vi "MIMIC Commands Rev 5.vi"(6 "MIMIC HOST COMMAND":T2(ring)=enum."Read Serial Number", 8 "Input String Data Array":string[](array[string])=["1"], 9 "HWHSflag":bool, 10 "wait (ms)":u32=500, 11 "VISA resource name":refnum<visa-resource-name>="COM5") -> (0 "error out":errorcluster={"status"=FALSE, "code"=1073676294, "source"="VISA Read in MIMIC RecvCommand.vi->MIMIC Commands Rev 2.vi"}, 1 "Receive_buffer":u8[](array[numeric]) format="%x", 2 "Receive_Unpacked_Data":T1)   [LabVIEW 2014]
panel:
  out "GUID":string
  out "Array":u8[](array[numeric])
  out "TimeToDecode":u16
  out "VISA resource name OUT":refnum<visa-resource-name>="COM5"
  out "hex integer string":string[](array[string])=["4", "D0", "0", "0", "FF", "2C"]
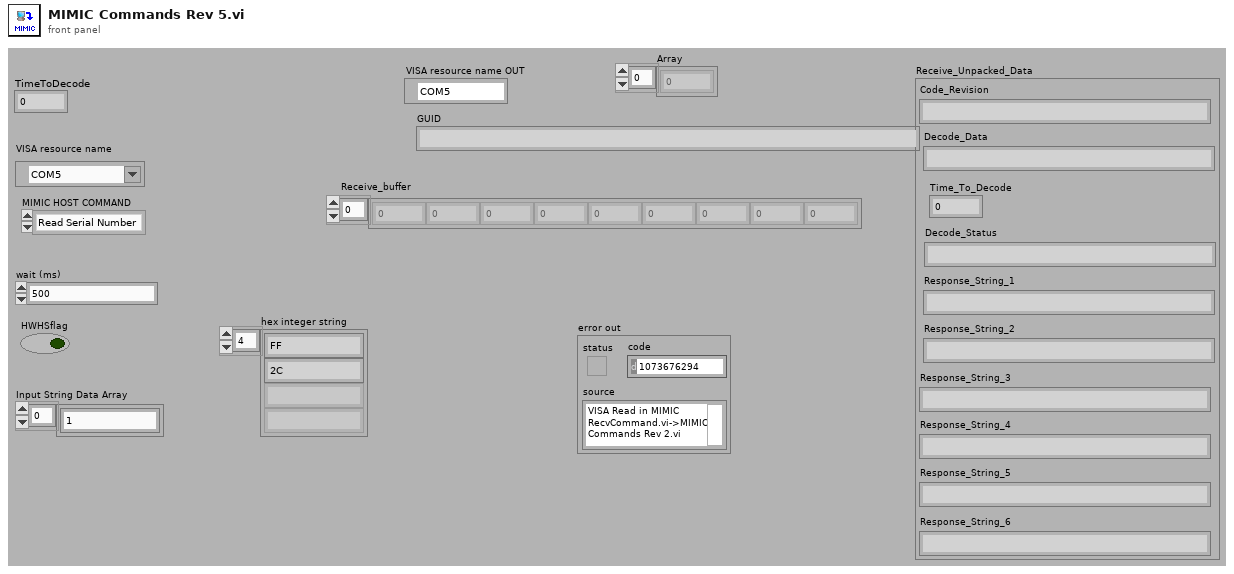
[diagram p1: front panel]
types:
  T1 = cluster{"Code_Revision":string, "Decode_Data":string, "Decode_Status":string, "Response_String_1":string, "Response_String_2":string, "Response_String_3":string, "Response_String_4":string, "Response_String_5":string, "Response_String_6":string, "Time_To_Decode":u16}
  T2 = enum16{"Enter FAT", "Beeper Control", "LED Off", "LED On", "Image Mode", "Start Session", "Stop Session", "Change Buadrate", "Auto Exposure", "Set Manual Exposure", "Read BT Address", "Store BT Address", "Pairing Command", "Query Paired Address", "Pairing Status", "Un-Pairing", "Set Illumination", "Trigger", "Set Defaults", "Imager Time To Decode Test", "Battery Off", "Battery Charge Control", "Read Battery Voltage", "Read Battery Temperature", "Software Version", "StoreFeatureSet", "ReadFeatureSet", "Store Model Number", "Read Model Number", "Store Manufacturing Date", "Read Manufacturing Date", "Store Service Date", "Read Service Date", "Store Serial Number", "Read Serial Number", "Exit FAT", "Read GUID", "Cable Auto ID", "Store RSM 627", "Read RSM 627", "Hall Effect switch", "Store GUID ", "Param Send"}
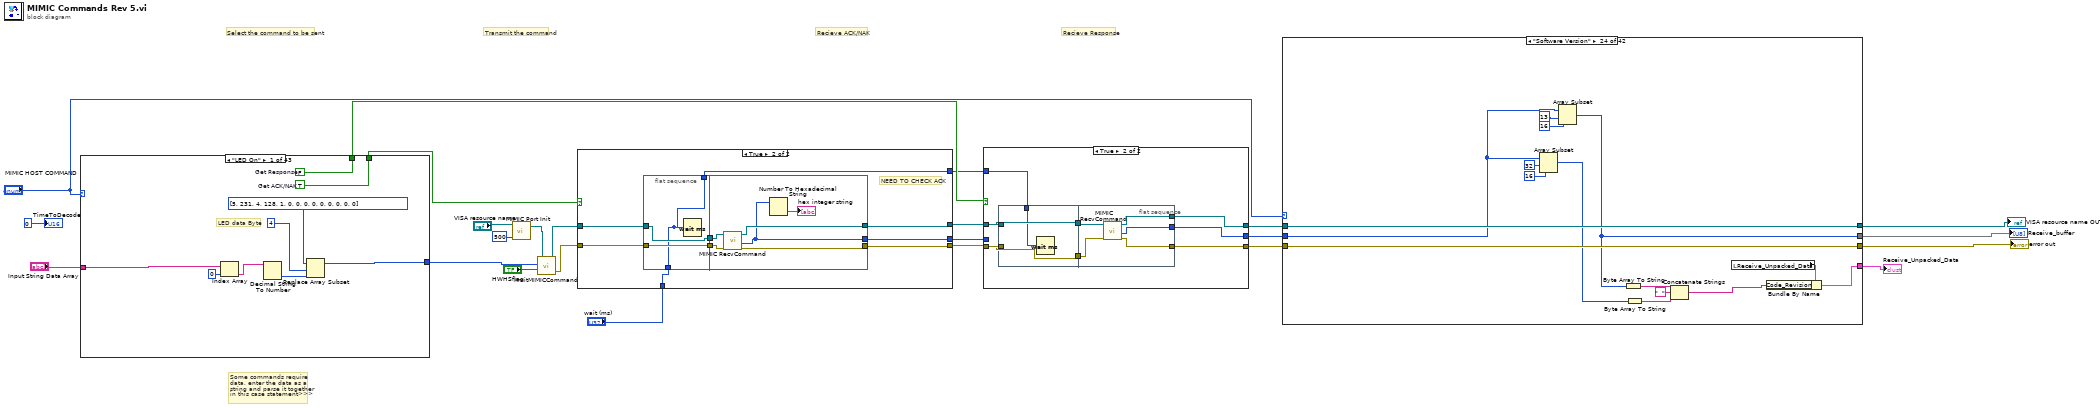
[diagram p0: block diagram]
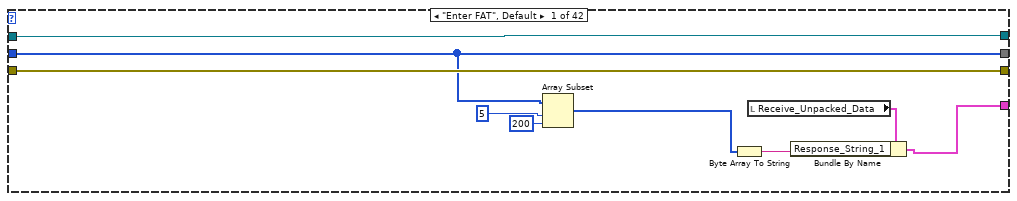
[diagram p2: hidden frame]
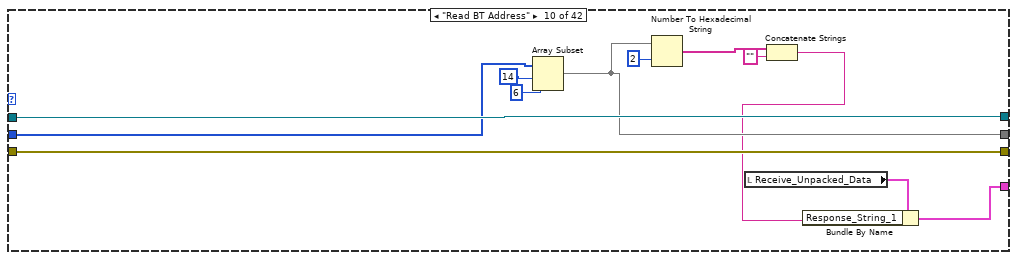
[diagram p11: hidden frame]
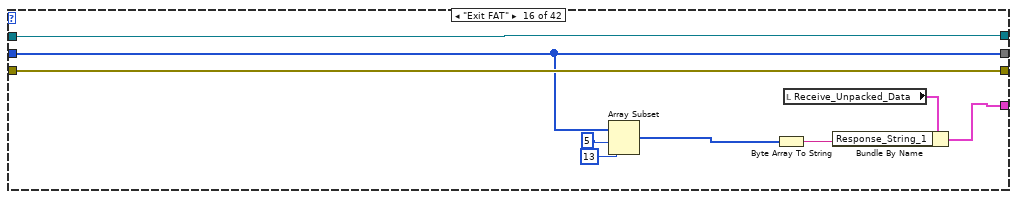
[diagram p17: hidden frame]
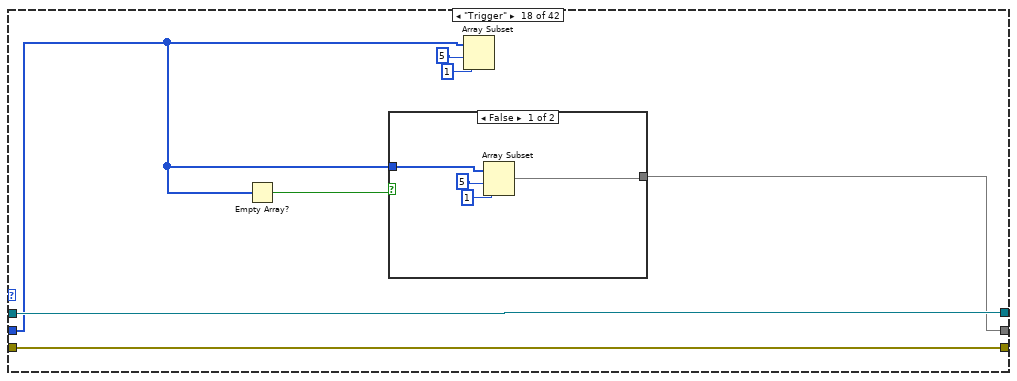
[diagram p19: hidden frame]
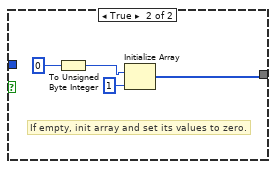
[diagram p20: hidden frame]
diagram:
  # "Transmit the command"
  # "Recieve Response"
  # "Recieve ACK/NAK"
  # "Select the command to be sent"
  # "Some commands require\ndata, enter the data as a\nstring and parse it together\nin this case statement>>>"
  n1 = case shown="\"LED On\"" "MIMIC HOST COMMAND" {
    tunnel: "Input String Data Array" -> [w33 w34 _ w45 _ _ _ w63 w79 w89 w104 w117 _ _ _ _ _ w141 _ _ _ w161 _ _ _ w178 _ w188 _ _ _ w214 _ w226 _ _ _ _ _ _ _ _ _]
    tunnel: [w27 w38 u8[] [5, 161, 4, 128, 16, 0, 0, 0, 0, 0, 0, 0, 0, 0] w46 u8[] [4, 228, 4, 0, 0, 0, 0, 0, 0, 0, 0, 0, 0, 0] u8[] [4, 228, 4, 0, 0, 0, 0, 0, 0, 0, 0, 0, 0, 0] u8[] [7, 215, 4, 0, 4, 11, 0, 255, 15, 0, 0, 0, 0, 0] w64 w73 w87 w102 w116 u8[] [16, 161, 4, 128, 16, 0, 0, 0, 0, 0, 0, 0, 0, 0] u8[] [5, 161, 4, 128, 16, 0, 0, 0, 0, 0, 0, 0, 0, 0] u8[] [4, 200, 4, 128, 0, 0, 0, 0, 0, 0, 0, 0, 0, 0] u8[] [5, 161, 4, 128, 25, 0, 0, 0, 0, 0, 0, 0, 0, 0] u8[] [7, 161, 4, 128, 66, 2, 29, 0, 0, 0, 0, 0, 0, 0] w140 u8[] [6, 161, 4, 128, 45, 2, 0, 0, 0, 0, 0, 0, 0, 0] u8[] [7, 161, 4, 128, 48, 19, 136, 0, 0, 0, 0, 0, 0, 0] u8[] [5, 161, 4, 128, 60, 0, 0, 0, 0, 0, 0, 0, 0, 0] w160 u8[] [7, 161, 4, 128, 66, 117, 48, 0, 0, 0, 0, 0, 0, 0] u8[] [7, 161, 4, 128, 66, 117, 49, 0, 0, 0, 0, 0, 0, 0] u8[] [7, 161, 4, 128, 66, 78, 41, 0, 0, 0, 0, 0, 0, 0] w180 u8[] [7, 161, 4, 128, 66, 2, 194, 0, 0, 0, 0, 0, 0, 0] w193 u8[] [7, 161, 4, 128, 66, 2, 21, 0, 0, 0, 0, 0, 0, 0] w207 u8[] [7, 161, 4, 128, 66, 2, 23, 0, 0, 0, 0, 0, 0, 0] w219 u8[] [7, 161, 4, 128, 66, 2, 24, 0, 0, 0, 0, 0, 0, 0] w231 u8[] [7, 161, 4, 128, 66, 2, 22, 0, 0, 0, 0, 0, 0, 0] u8[] [5, 161, 4, 128, 54, 254, 160, 0, 0, 0, 0, 0, 0, 0] u8[] [5, 161, 4, 128, 84, 0, 0, 0, 0, 0, 0, 0, 0, 0] u8[] [5, 161, 4, 128, 47] w246 u8[] [5, 161, 4, 128, 110] u8[] [10, 161, 4, 128, 69, 2, 115, 66, 7, 2] u8[] [6, 161, 4, 128, 45, 1, 0, 0, 0, 0, 0, 0, 0, 0] u8[] [7, 161, 4, 128, 66, 2, 115]] -> w19
    tunnel: [w26 w36 w43 w47 w55 w58 w60 w65 w80 w90 w105 w123 w126 w128 w131 w135 w139 w143 w150 w154 w157 w158 w169 w172 w174 w183 w186 w192 w197 w206 w211 w218 w222 w229 w234 w238 w242 w243 w251 w253 w256 w259 w263] -> w21
    tunnel: [w25 w37 w42 w48 w56 w59 w61 w66 w81 w91 w106 w124 w127 w129 w132 w134 w138 w142 w151 w153 w156 w159 w168 w171 w173 w182 w185 w191 w198 w205 w210 w217 w223 w230 w235 w237 w241 w244 w252 w254 w257 w260 w262] -> w23
    frame "LED On" {
      w26 = FALSE  # Get Response
      w25 = TRUE  # Get ACK/NAK
      # "LED data Byte"
      n2 = Index Array(array=w33, index=0) -> (element=w32:string)
      n3 = Decimal String To Number(string=w32) -> (number=w31:i32)  [unwired: 2 in, 1 out]
      n4 = Replace Array Subset(array=u8[] [5, 231, 4, 128, 1, 0, 0, 0, 0, 0, 0, 0, 0, 0], new element=w31, index=4) -> (w27:u8[])
    }
    frame "Beeper Control" {
      w36 = FALSE  # Get Response
      w37 = FALSE  # Get ACK/NAK
      # "Beeper data Byte"
      n5 = Decimal String To Number(string=w34, offset=0) -> (number=w41:i32[])  [unwired: 1 in, 1 out]
      n6 = Replace Array Subset(array=u8[] [5, 230, 4, 128, 0, 0, 0, 0, 0, 0, 0, 0, 0, 0], new element=w41, index=4) -> (w38:u8[])
    }
    frame "Enter FAT" {
      w43 = TRUE  # Get Response
      w42 = TRUE  # Get ACK/NAK
      # "Enter FAT command:\n0x05:0xA1:0x40:0x80:0x10"
    }
    frame "Image Mode" {
      w47 = FALSE  # Get Response
      w48 = TRUE  # Get ACK/NAK
      # "Image Mode Byte:\n00: Decode\n01: SnapShot\n02: Video\n03: Last Decode\n04: las No Decode"
      n7 = Index Array(array=w45, index=0) -> (element=w53:string)
      n8 = Decimal String To Number(string=w53) -> (number=w52:i32)  [unwired: 2 in, 1 out]
      n9 = Replace Array Subset(array=u8[] [5, 247, 4, 128, 0, 0, 0, 0, 0, 0, 0, 0, 0, 0], new element=w52, index=4) -> (w46:u8[])
    }
    frame "Start Session" {
      w55 = FALSE  # Get Response
      w56 = TRUE  # Get ACK/NAK
      # "Start Session"
    }
    frame "Stop Session" {
      w58 = FALSE  # Get Response
      w59 = TRUE  # Get ACK/NAK
      # "Start Session"
    }
    frame "Change Buadrate" {
      w60 = FALSE  # Get Response
      w61 = FALSE  # Get ACK/NAK
      # "Enter FAT command:\n06: 9600\n08: 38400\n0A: 57600\n0B:115200\n0C:230400"
    }
    frame "Auto Exposure" {
      w65 = FALSE  # Get Response
      w66 = TRUE  # Get ACK/NAK
      # "Auto Exposure:\n00:Disabled\n01: Enabled"
      n10 = Index Array(array=w63, index=0) -> (element=w71:string)
      n11 = Decimal String To Number(string=w71) -> (number=w70:i32)  [unwired: 2 in, 1 out]
      n12 = Replace Array Subset(array=u8[] [8, 198, 4, 0, 255, 240, 41, 0, 0, 0, 0, 0, 0, 0], new element=w70, index=7) -> (w64:u8[])
    }
    frame "Set Manual Exposure" {
      w80 = FALSE  # Get Response
      w81 = TRUE  # Get ACK/NAK
      # "Image Mode Byte:\n00: Decode\n01: SnapShot\n02: Video\n03: Last Decode\n04: las No Decode"
      n13 = Index Array(array=w79, index=0) -> (element=w85:string)
      n14 = Decimal String To Number(string=w85, default (0L)=u16 0 ("default (0 I32)")) -> (number=w78:u16)  [unwired: 1 in, 1 out]
      n15 = Split Number(x=w78) -> (hi(x)=w76:u8, lo(x)=w75:u8)
      n16 = Replace Array Subset(array=u8[] [10, 198, 4, 0, 255, 244, 241, 55, 0, 0, 0, 0, 0, 0], new element=w76, index=8) -> (w72:u8[])
      n17 = Replace Array Subset(array=w72, new element=w75, index=9) -> (w73:u8[])
    }
    frame "Store BT Address" {
      w90 = FALSE  # Get Response
      w91 = TRUE  # Get ACK/NAK
      # "Store BT command:\n0x16, 0xA1, 0x04, 0x80, 0x45, 0x02, 0x1D, 0x41, 0x07, 0x42, 0x00, 0x06, 0x00, 0x00, \n\t\t\t\t\t\t\t\t\t\t0x00, 0x00, 0x00, 0x00, 0x00, 0x00,0x00, 0x00, 0xFF, 0xFF};"
      n18 = for {
        N: 6 -> [_]
        tunnel: w89 -> [w100]
        tunnel: [w95] -> w87
        i -> [w97]
        n19 = Index Array(array=w100, index=w97) -> (element=w94:string)
        n20 = Add(x=14 ("index"), y=w97) -> (x+y=w98:i32)
        n21 = Hexadecimal String To Number(string=w94, offset=0) -> (number=w92:u32)  [unwired: 1 in, 1 out]
        n22 = local read "Array"() -> (w96:u8[])
        n23 = Replace Array Subset(array=w96, new element=w92, index=w98) -> (w95:u8[])
        n24 = local write "Array"(w95) -> ()
      }
      "Array" <- u8[] [22, 161, 4, 128, 69, 2, 29, 65, 7, 66, 0, 6, 0, 0, 0, 0, 0, 0, 0, 0, 255, 255, 255, 0, 0, 0]
    }
    frame "Param Send" {
      w105 = FALSE  # Get Response
      w106 = TRUE  # Get ACK/NAK
      # "Store BT command:\n0x16, 0xA1, 0x04, 0x80, 0x45, 0x02, 0x1D, 0x41, 0x07, 0x42, 0x00, 0x06, 0x00, 0x00, \n\t\t\t\t\t\t\t\t\t\t0x00, 0x00, 0x00, 0x00, 0x00, 0x00,0x00, 0x00, 0xFF, 0xFF};"
      n25 = for {
        N: 6 -> [_]
        tunnel: w104 -> [w115]
        tunnel: [w110] -> w102
        i -> [w112]
        n26 = Index Array(array=w115, index=w112) -> (element=w109:string)
        n27 = Add(x=14 ("index"), y=w112) -> (x+y=w113:i32)
        n28 = Hexadecimal String To Number(string=w109, offset=0) -> (number=w107:u32)  [unwired: 1 in, 1 out]
        n29 = local read "Array"() -> (w111:u8[])
        n30 = Replace Array Subset(array=w111, new element=w107, index=w113) -> (w110:u8[])
        n31 = local write "Array"(w110) -> ()
      }
      n32 = local write "Array"(u8[] [22, 161, 4, 128, 69, 2, 29, 65, 7, 66, 0, 6, 0, 0, 0, 0, 0, 0, 0, 0, 255, 255, 255, 0, 0, 0]) -> ()
    }
    frame "Pairing Command" {
      w123 = TRUE  # Get Response
      w124 = FALSE  # Get ACK/NAK
      # "Pairing  command:\n10 9E 04 80 00 00 02 03 06 08  01 0B 03 00 0F 0F FE 8E"
      n33 = Index Array(array=w117, index=0) -> (element=w121:string)
      n34 = String To Byte Array(string=w121) -> (unsigned byte array=w119:u8[])
      n35 = Replace Array Subset(array=u8[] [16, 158, 4, 128, 0, 0, 0, 0, 0, 8, 1, 11, 3, 0, 15, 15], new element=w119, index=4) -> (w116:u8[])
    }
    frame "Un-Pairing" {
      w126 = TRUE  # Get Response
      w127 = FALSE  # Get ACK/NAK
      # "Enter FAT command:\n0x05:0xA1:0x40:0x80:0x10"
    }
    frame "Set Illumination" {
      w128 = TRUE  # Get Response
      w129 = FALSE  # Get ACK/NAK
      # "Enter FAT command:\n0x05:0xA1:0x40:0x80:0x10"
    }
    frame "Set Defaults" {
      w131 = FALSE  # Get Response
      w132 = TRUE  # Get ACK/NAK
    }
    frame "Exit FAT" {
      w135 = TRUE  # Get Response
      w134 = TRUE  # Get ACK/NAK
    }
    frame "Read BT Address" {
      w139 = TRUE  # Get Response
      w138 = FALSE  # Get ACK/NAK
    }
    frame "LED Off" {
      w143 = FALSE  # Get Response
      w142 = TRUE  # Get ACK/NAK
      # "LED data Byte"
      n36 = Index Array(array=w141, index=0) -> (element=w148:string)
      n37 = Decimal String To Number(string=w148) -> (number=w147:i32)  [unwired: 2 in, 1 out]
      n38 = Replace Array Subset(array=u8[] [5, 232, 4, 128, 1, 0, 0, 0, 0, 0, 0, 0, 0, 0], new element=w147, index=4) -> (w140:u8[])
    }
    frame "Trigger" {
      w150 = TRUE  # Get Response
      w151 = TRUE  # Get ACK/NAK
    }
    frame "Imager Time To Decode Test" {
      w154 = TRUE  # Get Response
      w153 = TRUE  # Get ACK/NAK
      # "Start Session"
    }
    frame "Battery Off" {
      w157 = FALSE  # Get Response
      w156 = TRUE  # Get ACK/NAK
      # "Enter FAT command:\n0x05:0xA1:0x40:0x80:0x10"
    }
    frame "Battery Charge Control" {
      w158 = FALSE  # Get Response
      w159 = TRUE  # Get ACK/NAK
      # "Battery Charge\n0x06, 0xA1, 0x04, 0x80, 0x3D\n0x00: Disable charging of battery\n0x01: Enable charging of battery\n0x02: Enable Slow charge (Hammer)"
      n39 = Index Array(array=w161, index=0) -> (element=w166:string)
      n40 = Decimal String To Number(string=w166) -> (number=w165:i32)  [unwired: 2 in, 1 out]
      n41 = Replace Array Subset(array=u8[] [6, 161, 4, 128, 61, 0, 0, 0, 0, 0, 0, 0, 0, 0], new element=w165, index=5) -> (w160:u8[])
    }
    frame "Read Battery Voltage" {
      w169 = TRUE  # Get Response
      w168 = FALSE  # Get ACK/NAK
      # "Read Battery Voltage command:\n0x07:0xA1:0x04:0x80:0x42:0x75:0x30"
    }
    frame "Read Battery Temperature" {
      w172 = TRUE  # Get Response
      w171 = FALSE  # Get ACK/NAK
      # "Read Battery Temperature command:\n0x07:0xA1:0x04:0x80:0x42:0x75:0x31"
    }
    frame "Software Version" {
      w174 = TRUE  # Get Response
      w173 = TRUE  # Get ACK/NAK
      # "Software Version command:\n\"0x07, 0xA1, 0x04, 0x80, 0x42, 0x4E, 0x29,\""
    }
    frame "StoreFeatureSet" {
      w183 = FALSE  # Get Response
      w182 = TRUE  # Get ACK/NAK
      # "Store Feature Set command:\n\"0x0A, 0xA1, 0x04, 0x80, 0x45, 0x02, 0xC2, 0x42, 0x07,\n0xFF,//Feature Set Value \n0x00, 0x00}; //checksum\""
      n42 = Hexadecimal String To Number(string=w178, offset=0) -> (number=w176:u32[])  [unwired: 1 in, 1 out]
      n43 = Replace Array Subset(array=u8[] [10, 161, 4, 128, 69, 2, 194, 66, 7, 0, 0, 0, 0, 0], new element=w176, index=9) -> (w180:u8[])
    }
    frame "ReadFeatureSet" {
      w186 = TRUE  # Get Response
      w185 = TRUE  # Get ACK/NAK
      # "0x07, 0xA1, 0x04, 0x80, 0x42, 0x02, 0xC2, 0x00, 0x00};"
      # "Read Feature Set command:\n0x07, 0xA1, 0x04, 0x80, 0x42, 0x02, 0xC2,"
    }
    frame "Store Model Number" {
      w192 = FALSE  # Get Response
      w191 = TRUE  # Get ACK/NAK
      # "StoreModel Number command:\n0x20, 0xA1, 0x04, 0x80, 0x45, 0x02, 0x15, 0x53, 0x07, 0x00, 0x12, 0x00, 0x00,\n\t\t\t\t\t\t\t\t\t\t0x00, 0x00, 0x00, 0x00, 0x00, 0x00, 0x00, 0x00, 0x00,\n\t\t\t\t\t\t\t\t\t\t0x00, 0x00, 0x00, 0x00, 0x00, 0x00, 0x00, 0x00, 0x00,\n\t\t\t\t\t\t\t\t\t\t0x00"
      n44 = Index Array(array=w188, index=0) -> (element=w189:string)
      n45 = String To Byte Array(string=w189) -> (unsigned byte array=w190:u8[])
      n46 = Replace Array Subset(array=u8[] [32, 161, 4, 128, 69, 2, 21, 83, 7, 0, 18, 0, 0, 0, 0, 0, 0, 0, 0, 0, 0, 0, 0, 0, 0, 0, 0, 0, 0, 0, 0, 0, 0], new element=w190, index=13) -> (w193:u8[])
    }
    frame "Read Model Number" {
      w197 = TRUE  # Get Response
      w198 = TRUE  # Get ACK/NAK
      # "ReadModel Number command:\n0x07, 0xA1, 0x04, 0x80, 0x42, 0x02, 0x15,"
    }
    frame "Store Manufacturing Date" {
      w206 = FALSE  # Get Response
      w205 = TRUE  # Get ACK/NAK
      # "Store Manufacturing Date command:\n0x15, 0xA1, 0x04, 0x80, 0x45, 0x02, 0x17, 0x53, 0x07, 0x00, 0x07, 0x00, 0x00,\n\t\t\t\t\t\t\t\t\t\t0x00, 0x00, 0x00, 0x00, 0x00, 0x00, 0x00,\n\t\t\t\t\t\t\t\t\t\t0x00"
      n47 = Get Date/Time In Seconds() -> (seconds since 1Jan1904=w204:timestamp)
      n48 = Format Date/Time String(time format string (%c)="%d%b%y", seconds (now)=w204, UTC format=FALSE) -> (date/time string=w200:string)
      n49 = To Upper Case(1:w200) -> (0:w199:string)
      n50 = String To Byte Array(string=w199) -> (unsigned byte array=w201:u8[])
      n51 = Replace Array Subset(array=u8[] [21, 161, 4, 128, 69, 2, 23, 83, 7, 0, 7, 0, 0, 0, 0, 0, 0, 0, 0, 0, 0, 0], new element=w201, index=13) -> (w207:u8[])
    }
    frame "Read Manufacturing Date" {
      w211 = TRUE  # Get Response
      w210 = TRUE  # Get ACK/NAK
      # "Read Feature Set command:\n0x07, 0xA1, 0x04, 0x80, 0x42, 0x02, 0x17,"
    }
    frame "Store Service Date" {
      w218 = FALSE  # Get Response
      w217 = TRUE  # Get ACK/NAK
      # "StoreService Date command:\n0x15, 0xA1, 0x04, 0x80, 0x45, 0x02, 0x18, 0x53, 0x07, 0x00, 0x07, 0x00, 0x00,\n\t\t\t\t\t\t\t\t\t\t0x00, 0x00, 0x00, 0x00, 0x00, 0x00, 0x00,\n\t\t\t\t\t\t\t\t\t\t0x00"
      n52 = Index Array(array=w214, index=0) -> (element=w216:string)
      n53 = String To Byte Array(string=w216) -> (unsigned byte array=w213:u8[])
      n54 = Replace Array Subset(array=u8[] [21, 161, 4, 128, 69, 2, 24, 83, 7, 0, 7, 0, 0, 0, 0, 0, 0, 0, 0, 0, 0, 0], new element=w213, index=13) -> (w219:u8[])
    }
    frame "Read Service Date" {
      w222 = TRUE  # Get Response
      w223 = TRUE  # Get ACK/NAK
      # "Read Service Date command:\n0x07, 0xA1, 0x04, 0x80, 0x42, 0x02, 0x18,"
    }
    frame "Store Serial Number" {
      w229 = FALSE  # Get Response
      w230 = TRUE  # Get ACK/NAK
      # "Store Serial Number command:\n0x1E, 0xA1, 0x04, 0x80, 0x45, 0x02, 0x16, 0x53, 0x07, 0x00, 0x10, 0x00, 0x00,\n\t\t\t\t\t\t\t\t\t\t0x00, 0x00, 0x00, 0x00, 0x00, 0x00, 0x00, 0x00,\n\t\t\t\t\t\t\t\t\t\t0x00, 0x00, 0x00, 0x00, 0x00, 0x00, 0x00, 0x00,\n\t\t\t\t\t\t\t\t\t\t0x00"
      n55 = Index Array(array=w226, index=0) -> (element=w228:string)
      n56 = String To Byte Array(string=w228) -> (unsigned byte array=w225:u8[])
      n57 = Replace Array Subset(array=u8[] [30, 161, 4, 128, 69, 2, 22, 83, 7, 0, 16, 0, 0, 0, 0, 0, 0, 0, 0, 0, 0, 0, 0, 0, 0, 0, 0, 0, 0, 0, 0, 0, 0], new element=w225, index=13) -> (w231:u8[])
    }
    frame "Read Serial Number" {
      w234 = TRUE  # Get Response
      w235 = TRUE  # Get ACK/NAK
      # "Read Serial Number command:\n0x07, 0xA1, 0x04, 0x80, 0x42, 0x02, 0x16,"
    }
    frame "Pairing Status" {
      w238 = TRUE  # Get Response
      w237 = FALSE  # Get ACK/NAK
      # "Read Serial Number command:\n0x05, 0xA1, 0x04, 0x80, 0x36, 0xFE, 0xA0,"
    }
    frame "Query Paired Address" {
      w242 = TRUE  # Get Response
      w241 = FALSE  # Get ACK/NAK
      # "Read Serial Number command:\n0x05, 0xA1, 0x04, 0x80, 0x54,"
    }
    frame "Read GUID" {
      w243 = TRUE  # Get Response
      w244 = TRUE  # Get ACK/NAK
      # "\"0x05, 0xA1, 0x04, 0x80, 0x2F,\""
    }
    frame "Store GUID " {
      w251 = TRUE  # Get Response
      w252 = FALSE  # Get ACK/NAK
      # "32 bytes 0-9, A-F (0x30 - 0x3F, 0x41 - 0x46)"
      # "Start of Date Bytes"
      # "Store GIUD command:\n0x29:0x80:0x04:0x80:0x00:0x25:0x64:0x00:0x0B:0xXX:0xXX:0xXX:0xXX:0xXX:0xXX:0xXX:0xXX:0xXX:0xXX:0xXX:0xXX:0xXX:0xXX:0xXX:0xXX:0xXX:0xXX:0xXX:0xXX:0xXX:0xXX:0xXX:0xXX:0xXX:0xXX:0xXX:0xXX:0xXX:0xXX:0xXX:0xXX:"
      n58 = call "Generate GUID.vi"() -> ("GUID"=w250:string)  [unwired: 10 in, 1 out]
      "GUID" <- w250
      n59 = String To Byte Array(string=w250) -> (unsigned byte array=w247:u8[])
      n60 = Insert Into Array(array=u8[] [41, 128, 4, 128, 0, 37, 100, 0, 11], index=9, new element=w247) -> (w246:u8[])
    }
    frame "Cable Auto ID" {
      w253 = TRUE  # Get Response
      w254 = TRUE  # Get ACK/NAK
      # "0x05, 0xA1, 0x04, 0x00, 0x6E"
    }
    frame "Store RSM 627" {
      w256 = FALSE  # Get Response
      w257 = TRUE  # Get ACK/NAK
      # "0x0A, 0xA1, 0x04, 0x80, 0x45, 0x02, 0x73, 0x42, 0x07, 0x02"
    }
    frame "Hall Effect switch" {
      w259 = TRUE  # Get Response
      w260 = TRUE  # Get ACK/NAK
    }
    frame "Read RSM 627" {
      w263 = TRUE  # Get Response
      w262 = TRUE  # Get ACK/NAK
      # "\"0x07, 0xA1, 0x04, 0x80, 0x42,0x02,0x73\""
    }
  }
  n61 = call "MIMIC Port Init.vi"("MIMIC TIMEOUT"=u32 500, "MIMIC_PORT"="VISA resource name") -> ("MIMIC PORT RESOURCE"=w3:refnum<visa-resource-name>)  [unwired: 1 in, 1 out]
  n62 = call "XmitMIMICCommand.vi"("HWHSflag"="HWHSflag", "Command array"=w19, "VISA resource name"=w3) -> ("error out"=w17:errorcluster, "VISA resource name Out"=w16:refnum<visa-resource-name>)  [unwired: 1 in]
  n63 = case shown="True" w23 {
    tunnel: [w267 w271] -> w22
    tunnel: w17 -> [w267 w276]
    tunnel: w16 -> [w266 w274]
    tunnel: [w266 w272] -> w20
    tunnel: [_ w270] -> w11
    tunnel: [w265 w269] -> w10
    tunnel: "wait (ms)" -> [w265 w268]
    frame False {
    }
    frame True {
      # "NEED TO CHECK ACK"
      n64 = flat-sequence {
        tunnel: w276 -> [w279]
        tunnel: [w279] -> w275
        tunnel: w274 -> [w278]
        tunnel: [w278] -> w273
        tunnel: [w277] -> w269
        tunnel: w268 -> [w277]
        tunnel: w275 -> [w284]
        tunnel: w273 -> [w283]
        tunnel: [w282] -> w272
        tunnel: [w281] -> w271
        tunnel: [w280] -> w270
        frame #0 {
          n65 = Wait (ms)(milliseconds to wait=w277) -> ()  [unwired: 1 out]
        }
        frame #1 {
          n66 = call "MIMIC RecvCommand.vi"("error in"=w284, "VISA resource name"=w283) -> ("error out"=w281:errorcluster, "Receive_buffer"=w280:u8[], "VISA resource name OUT"=w282:refnum<visa-resource-name>)  [unwired: 2 in, 1 out]
          n67 = Number To Hexadecimal String(2:w280) -> (0:→"hex integer string":string[])  [unwired: 1 in]
        }
      }
    }
  }
  n68 = case shown="True" w21 {
    tunnel: [w288 w295] -> w12
    tunnel: w22 -> [w288 w290]
    tunnel: w20 -> [w287 w292]
    tunnel: [w286 w296] -> w13
    tunnel: [w287 w294] -> w14
    tunnel: w11 -> [w286 _]
    tunnel: w10 -> [_ w289]
    frame False {
    }
    frame True {
      n69 = flat-sequence {
        tunnel: [w299] -> w293
        tunnel: w292 -> [w299]
        tunnel: [w298] -> w291
        tunnel: w290 -> [w298]
        tunnel: w289 -> [w297]
        tunnel: [w304] -> w296
        tunnel: [w303] -> w295
        tunnel: [w302] -> w294
        tunnel: w293 -> [w300]
        tunnel: w291 -> [w301]
        frame #0 {
          n70 = Wait (ms)(milliseconds to wait=w297) -> ()  [unwired: 1 out]
        }
        frame #1 {
          n71 = call "MIMIC RecvCommand.vi"("error in"=w301, "VISA resource name"=w300) -> ("error out"=w303:errorcluster, "Receive_buffer"=w304:u8[], "VISA resource name OUT"=w302:refnum<visa-resource-name>)  [unwired: 2 in, 1 out]
        }
      }
    }
  }
  n72 = case shown="\"Software Version\"" "MIMIC HOST COMMAND" {
    tunnel: w14 -> [w312 w316 w319 w322 w325 w328 w331 w334 w337 w349 w352 w355 w358 w361 w364 w373 w376 w383 w402 w425 w428 w434 w436 w453 w458 w461 w465 w475 w486 w494 w497 w506 w508 w519 w530 w535 w553 w556 w559 w562 w567 w580]
    tunnel: [w312 w316 w319 w322 w325 w328 w331 w334 w337 w349 w352 w355 w358 w361 w364 w373 w376 w383 w402 w425 w428 w434 w436 w453 w458 w461 w465 w475 w486 w494 w497 w506 w508 w519 w530 w535 w553 w556 w559 w562 w567 w580] -> w8
    tunnel: w13 -> [w308 w315 w318 w321 w324 w327 w330 w333 w336 w347 w351 w354 w357 w360 w363 w365 w375 w378 w400 w424 w427 w430 w438 w448 w457 w462 w466 w472 w485 w491 w496 w503 w509 w515 w523 w532 w548 w555 w558 w561 w564 w579]
    tunnel: [w308 w315 w318 w321 w324 w327 w330 w333 w336 w342 w351 w354 w357 w360 w363 w365 w375 w377 w400 w424 w427 w429 w437 w451 w457 w459 w466 w470 w485 w488 w496 w501 w509 w511 w521 w534 w547 w555 w558 w561 w563 w579] -> w7
    tunnel: w12 -> [w313 w314 w317 w320 w323 w326 w329 w332 w335 w348 w350 w353 w356 w359 w362 w372 w374 w382 w403 w423 w426 w433 w435 w452 w456 w460 w467 w476 w484 w495 w498 w507 w510 w518 w531 w536 w552 w554 w557 w560 w566 w578]
    tunnel: [w313 w314 w317 w320 w323 w326 w329 w332 w335 w348 w350 w353 w356 w359 w362 w372 w374 w382 w403 w423 w426 w433 w435 w452 w456 w460 w467 w476 w484 w495 w498 w507 w510 w518 w531 w536 w552 w554 w557 w560 w566 w578] -> w6
    tunnel: [w310 _ _ _ _ _ _ _ _ w343 _ _ _ _ _ w369 _ _ w405 _ _ _ _ w449 _ _ _ w468 w478 w489 _ w499 _ w513 w522 _ w545 _ _ _ _ _] -> w4
    frame "Enter FAT", Default {
      n73 = Array Subset(array=w308, index=5, length=200) -> (w307:u8[])
      n74 = Byte Array To String(unsigned byte array=w307) -> (string=w311:string)
      n75 = local read "Receive_Unpacked_Data"() -> (w309:T1)
      n76 = Bundle By Name(cluster=w309, "Response_String_1"=w311) -> (w310:T1)
    }
    frame "Beeper Control" {
    }
    frame "LED On" {
    }
    frame "Image Mode" {
    }
    frame "Start Session" {
    }
    frame "Stop Session" {
    }
    frame "Change Buadrate" {
    }
    frame "Auto Exposure" {
    }
    frame "Set Manual Exposure" {
    }
    frame "Read BT Address" {
      n77 = Array Subset(array=w347, index=14, length=6) -> (w342:u8[])
      n78 = Number To Hexadecimal String(1:i16 2 ("width (-)"), 2:w342) -> (0:w340:string[])
      n79 = local read "Receive_Unpacked_Data"() -> (w344:T1)
      n80 = Concatenate Strings(w340, "" ("string")) -> (w339:string)
      n81 = Bundle By Name(cluster=w344, "Response_String_1"=w339) -> (w343:T1)
    }
    frame "Store BT Address" {
    }
    frame "Pairing Command" {
    }
    frame "Un-Pairing" {
    }
    frame "Set Illumination" {
    }
    frame "Set Defaults" {
    }
    frame "Exit FAT" {
      n82 = Array Subset(array=w365, index=5, length=13) -> (w366:u8[])
      n83 = Byte Array To String(unsigned byte array=w366) -> (string=w371:string)
      n84 = local read "Receive_Unpacked_Data"() -> (w370:T1)
      n85 = Bundle By Name(cluster=w370, "Response_String_1"=w371) -> (w369:T1)
    }
    frame "LED Off" {
    }
    frame "Trigger" {
      n86 = Empty Array?(array=w378) -> (empty?=w379:bool)
      n87 = case shown="False" w379 {
        tunnel: w378 -> [w385 _]
        tunnel: [w384 w391] -> w377
        frame False {
          n88 = Array Subset(array=w385, index=5, length=1) -> (w384:u8[])
        }
        frame True {
          # "If empty, init array and set its values to zero."
          n89 = To Unsigned Byte Integer(number=u8 0) -> (unsigned 8bit integer=w389:u8)
          n90 = Initialize Array(w389, 1 ("dimension size")) -> (w391:u8[])
        }
      }
      n91 = Array Subset(array=w378, index=5, length=1) -> ()  [unwired: 1 out]
    }
    frame "Imager Time To Decode Test" {
      n92 = Byte Array To String(unsigned byte array=w400) -> (string=w416:string)
      n93 = Replace Substring(2:17 ("length (len. of substring)"), 3:0 ("offset (0)"), 5:w416) -> (1:w411:string)  [unwired: 1 in, 1 out]
      n94 = String Length(string=w411) -> (length=w410:i32)
      n95 = Index Array(array=w400, index=5) -> (element=w413:u8)
      n96 = Subtract(x=w410, y=2) -> (x-y=w408:i32)
      n97 = Index Array(array=w400, index=7 ("length")) -> (element=w395:u8)
      n98 = Index Array(array=w400, index=6) -> (element=w398:u8)
      n99 = case shown="1" w413 {
        frame 0, Default {
          n100 = local read "Receive_Unpacked_Data"() -> (w417:T1)
          n101 = Bundle By Name(cluster=w417, "Decode_Status"="No Decode" ("Decode_Data")) -> (w418:T1)
          n102 = local write "Receive_Unpacked_Data"(w418) -> ()
        }
        frame 1 {
          n103 = local read "Receive_Unpacked_Data"() -> (w421:T1)
          n104 = Bundle By Name(cluster=w421, "Decode_Status"="SUCCESS" ("Decode_Data")) -> (w420:T1)
          n105 = local write "Receive_Unpacked_Data"(w420) -> ()
        }
      }
      n106 = Join Numbers(hi=u8 0, lo=w398) -> ((hi.lo)=w393:u16)
      n107 = Join Numbers(hi=w395, lo=u8 0 ("hi")) -> ((hi.lo)=w394:u16)
      n108 = Add(x=w393, y=w394) -> (x+y=w392:u16)
      n109 = local write "TimeToDecode"(w392) -> ()
      n110 = Replace Substring(2:2 ("length (len. of substring)"), 3:w408, 5:w411) -> (1:w406:string)  [unwired: 1 in, 1 out]
      n111 = local read "Receive_Unpacked_Data"() -> (w404:T1)
      n112 = Bundle By Name(cluster=w404, "Decode_Data"=w406, "Time_To_Decode"=w392) -> (w405:T1)
    }
    frame "Battery Off" {
    }
    frame "Battery Charge Control" {
    }
    frame "Read Battery Voltage" {
      # "Voltage (MSB_LSB *.0006*2)"
      # "RESPONSE\nLength Byte:\t0x0D\nOpcode Byte:\t0x21\nSource Byte:\t0x00\nStatus Byte:\t0x80\nSub-opcode Byte:\t0x42\nData Byte 1:\t0x75: Attribute MSB\nData Byte 2:\t0x30: Attribute LSB\nData Byte 3:\t0x57: Attribute is Word ('W') value\nData Byte 4:\t0x01\nData Byte 5:\t0xXX: Battery Voltage MSB\nData Byte 6:\t0xXX: Battery Voltage LSB\nData Byte 7:\t0xFF: Packet Termination\nData Byte 8:\t0xFF: Packet Termination\nChecksum High Byte:\t0xXX\nChecksum Low Byte:\t0xXX"
      n113 = Array Subset(array=w430, index=0, length=15) -> (w429:u8[])
    }
    frame "Read Battery Temperature" {
      # "RESPONSE\nLength Byte:\t0x0D\nOpcode Byte:\t0x21\nSource Byte:\t0x00\nStatus Byte:\t0x80\nSub-opcode Byte:\t0x42\nData Byte 1:\t0x75: Attribute MSB\nData Byte 2:\t0x31: Attribute LSB\nData Byte 3:\t0x57: Attribute is Word ('W') value\nData Byte 4:\t0x01\nData Byte 5:\t0xXX: Battery Temperature MSB\nData Byte 6:\t0xXX: Battery Temperature LSB\nData Byte 7:\t0xFF: Packet Termination\nData Byte 8:\t0xFF: Packet Termination\nChecksum High Byte:\t0xXX\nChecksum Low Byte:\t0xXX"
      n114 = Array Subset(array=w438, index=0, length=15) -> (w437:u8[])
    }
    frame "Software Version" {
      n115 = Array Subset(array=w448, index=32, length=16) -> (w445:u8[])
      n116 = Array Subset(array=w448, index=13, length=16) -> (w451:u8[])
      n117 = Byte Array To String(unsigned byte array=w451) -> (string=w444:string)
      n118 = Byte Array To String(unsigned byte array=w445) -> (string=w443:string)
      n119 = Concatenate Strings(w444, "  " ("string"), w443) -> (w441:string)
      n120 = local read "Receive_Unpacked_Data"() -> (w450:T1)
      n121 = Bundle By Name(cluster=w450, "Code_Revision"=w441) -> (w449:T1)
    }
    frame "StoreFeatureSet" {
    }
    frame "ReadFeatureSet" {
      # "Feature Set Responce:\n0x0C, 0x21, 0x00, 0x00, 0x42, 0x02, 0xC2,0x42,0x01,\n\t\t\t\t\t\t\t\t\t\t\t  \t\t\t  0xff, //FEATURE-SET\n\t\t\t\t\t\t\t\t\t\t\t\t\t\t  0xff,0xff, // packet termination\n\t\t\t\t\t\t\t\t\t\t\t\t\t\t  0x00, 0x00}; //checksum"
      n122 = Array Subset(array=w462, index=9, length=1) -> (w459:u8[])
    }
    frame "Store Model Number" {
    }
    frame "Read Model Number" {
      n123 = Array Subset(array=w472, index=13, length=18) -> (w470:u8[])
      n124 = Byte Array To String(unsigned byte array=w470) -> (string=w471:string)
      n125 = local read "Receive_Unpacked_Data"() -> (w469:T1)
      n126 = Bundle By Name(cluster=w469, "Response_String_1"=w471) -> (w468:T1)
    }
    frame "Store Manufacturing Date" {
      n127 = Get Date/Time In Seconds() -> (seconds since 1Jan1904=w483:timestamp)
      n128 = Format Date/Time String(time format string (%c)="%d%b%y", seconds (now)=w483, UTC format=FALSE) -> (date/time string=w480:string)
      n129 = To Upper Case(1:w480) -> (0:w477:string)
      n130 = local read "Receive_Unpacked_Data"() -> (w479:T1)
      n131 = Bundle By Name(cluster=w479, "Response_String_1"=w477) -> (w478:T1)
    }
    frame "Read Manufacturing Date" {
      n132 = Array Subset(array=w491, index=13, length=7) -> (w488:u8[])
      n133 = Byte Array To String(unsigned byte array=w488) -> (string=w490:string)
      n134 = local read "Receive_Unpacked_Data"() -> (w487:T1)
      n135 = Bundle By Name(cluster=w487, "Response_String_1"=w490) -> (w489:T1)
    }
    frame "Store Service Date" {
    }
    frame "Read Service Date" {
      n136 = Array Subset(array=w503, index=13, length=7) -> (w501:u8[])
      n137 = Byte Array To String(unsigned byte array=w501) -> (string=w502:string)
      n138 = local read "Receive_Unpacked_Data"() -> (w500:T1)
      n139 = Bundle By Name(cluster=w500, "Response_String_1"=w502) -> (w499:T1)
    }
    frame "Store Serial Number" {
    }
    frame "Read Serial Number" {
      n140 = Array Subset(array=w515, index=13, length=16) -> (w511:u8[])
      n141 = Byte Array To String(unsigned byte array=w511) -> (string=w514:string)
      n142 = local read "Receive_Unpacked_Data"() -> (w512:T1)
      n143 = Bundle By Name(cluster=w512, "Response_String_1"=w514) -> (w513:T1)
    }
    frame "Query Paired Address" {
      # "Cradle BT Address"
      # "Pair Status\n0x00: Unpaired \n0x01: Paired"
      n144 = Array Subset(array=w523, index=6, length=6) -> (w526:u8[])
      n145 = Array Subset(array=w523, index=5, length=1) -> (w521:u8[])
      n146 = local read "Receive_Unpacked_Data"() -> (w520:T1)
      n147 = Byte Array To String(unsigned byte array=w526) -> (string=w527:string)
      n148 = Bundle By Name(cluster=w520, "Response_String_1"=w527) -> (w522:T1)
    }
    frame "Pairing Status" {
      # "Pairing Status\n0x00: Cradle is not paired\n0x01: Cradle is paired"
      n149 = Empty Array?(array=w532) -> (empty?=w533:bool)
      n150 = case shown="False" w533 {
        tunnel: w532 -> [w538 _]
        tunnel: [w537 w544] -> w534
        frame False {
          n151 = Array Subset(array=w538, index=5, length=1) -> (w537:u8[])
        }
        frame True {
          # "If empty, init array and set its values to zero."
          n152 = To Unsigned Byte Integer(number=u8 0) -> (unsigned 8bit integer=w542:u8)
          n153 = Initialize Array(w542, 1 ("dimension size")) -> (w544:u8[])
        }
      }
    }
    frame "Read GUID" {
      n154 = Array Subset(array=w548, index=5, length=32) -> (w547:u8[])
      n155 = Byte Array To String(unsigned byte array=w547) -> (string=w551:string)
      n156 = local read "Receive_Unpacked_Data"() -> (w546:T1)
      n157 = Bundle By Name(cluster=w546, "Response_String_1"=w551) -> (w545:T1)
    }
    frame "Cable Auto ID" {
    }
    frame "Store RSM 627" {
    }
    frame "Store GUID " {
    }
    frame "Hall Effect switch" {
      n158 = Empty Array?(array=w564) -> (empty?=w565:bool)
      n159 = case shown="True" w565 {
        tunnel: w564 -> [w571 _]
        tunnel: [w570 w577] -> w563
        frame False {
          n160 = Array Subset(array=w571, index=5, length=1) -> (w570:u8[])
        }
        frame True {
          # "If empty, init array and set its values to zero."
          n161 = To Unsigned Byte Integer(number=u8 0) -> (unsigned 8bit integer=w575:u8)
          n162 = Initialize Array(w575, 1 ("dimension size")) -> (w577:u8[])
        }
      }
      n163 = Array Subset(array=w564, index=5, length=1) -> ()  [unwired: 1 out]
    }
    frame "Read RSM 627" {
    }
  }
  "error out" <- w6
  "Receive_buffer" <- w7
  "VISA resource name OUT" <- w8
  "Receive_Unpacked_Data" <- w4
  "TimeToDecode" <- u16 0 ("TimeToDecode")
